vi "PH_gentec_Powermeter.PC Set Statistics Config.vi"(0 "VI in":refnum<vi>, 2 "Data Sampling Settings":T1={"Sample Rate"=0, "Sample Rate Unit"=1, "Sample Period"=0, "Sample Period Unit"=0, "Total Duration"=0, "Total Duration Unit"=0, "Time Stamp"=0} {"Time Stamp" items=["Off", "On"]; "Total Duration Unit" items=["Period", "Seconds", "Minutes", "Hours", "Days", "Weeks", "Continuous", "# of Points"]; "Total Duration" max=300 step=1; "Sample Period Unit" items=["Seconds", "Minutes", "Hours", "Days", "Weeks", "Pulses"]; "Sample Rate Unit" items=["per Second", "per Minute", "per Hour", "per Day", "% pulses"]; "Sample Rate" max=300 step=1}, 5 "error in (no error)":errorcluster) -> (14 "VI out":refnum<vi>, 19 "error out":errorcluster)   [LabVIEW 2014, in "PH_gentec_Powermeter.lvlib"]
uses:
  PH_gentec_Powermeter.lvlib
  instr.lib/gentec-SOLO-PE/Driver/Type Defs/gentec-SOLO-PE.Data Sampling Settings.ctl
  instr.lib/gentec-SOLO-PE/gentec-SOLO-PE - Driver.lvlib
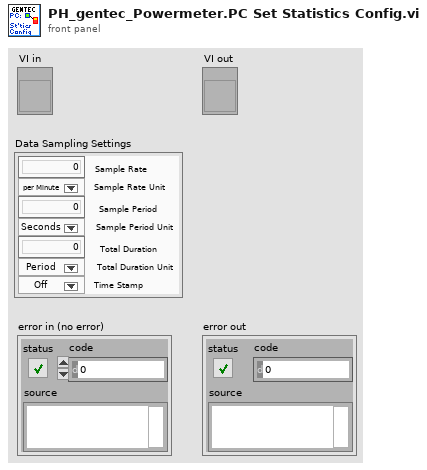
[diagram p1: front panel]
types:
  T1 = typedef "gentec-SOLO-PE - Driver.lvlib/gentec-SOLO-PE.Data Sampling Settings.ctl" = cluster{"Sample Rate":u32, "Sample Rate Unit":u32, "Sample Period":u32, "Sample Period Unit":u32, "Total Duration":u32, "Total Duration Unit":u32, "Time Stamp":u32}
  T2 = typedef "PH_gentec_Powermeter.lvlib/PH_gentec_Powermeter.i attribute.ctl" = cluster{"GUI References":cluster{"delete":refnum<vi>, "start stop Statistics":refnum<vi>, "Statistic Data":refnum<vi>, "Configuration Values":refnum<vi>, "Set Zero":refnum<vi>, "Data Sampling Settings":refnum<vi>, "Wanted Sets":refnum<vi>, "Current Sets":refnum<vi>}, "Start Stop Statistics":bool, "Wanted Sets":T3, "Current Sets":T3}
  T3 = typedef "PH_gentec_Powermeter.lvlib/PH_gentec_Powermeter.Sets.ctl" = cluster{"Data Sampling Settings":T1, "Set Zero":bool}
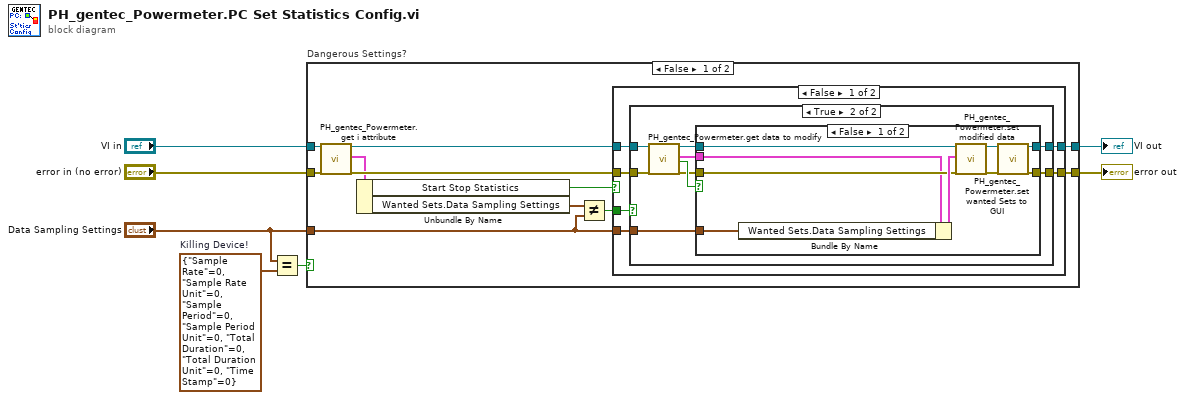
[diagram p0: block diagram]
diagram:
  w2 = T1 {"Sample Rate"=0, "Sample Rate Unit"=0, "Sample Period"=0, "Sample Period Unit"=0, "Total Duration"=0, "Total Duration Unit"=0, "Time Stamp"=0}  # Killing Device!
  n1 = Equal?(x="Data Sampling Settings", y=w2) -> (x = y?=w1:bool)
  n2 = case "Dangerous Settings?" shown="False" w1 {
    tunnel: "error in (no error)" -> [w18 w49]
    tunnel: "VI in" -> [w16 w50]
    tunnel: [w10 w50] -> w5
    tunnel: [w9 w49] -> w4
    tunnel: "Data Sampling Settings" -> [w8 _]
    frame False {
      n3 = call "PH_gentec_Powermeter.get i attribute.vi"("i ref in"=w16, "error in (no error)"=w18) -> ("i ref out"=w15:refnum<vi>, "i attribute"=w14:T2, "error out"=w17:errorcluster)  [unwired: 15 in]
      n4 = Unbundle By Name(w14) -> ("Start Stop Statistics"=w11:bool, "Wanted Sets.Data Sampling Settings"=w13:T1)
      n5 = Not Equal?(x=w13, y=w8) -> (x != y?=w12:bool)
      n6 = case shown="False" w11 {
        tunnel: w17 -> [w24 w47]
        tunnel: w15 -> [w23 w48]
        tunnel: w8 -> [w22 _]
        tunnel: w12 -> [w21 _]
        tunnel: [w20 w48] -> w10
        tunnel: [w19 w47] -> w9
        frame False {
          n7 = case shown="True" w21 {
            tunnel: [w25 w35] -> w19
            tunnel: [w26 w34] -> w20
            tunnel: w24 -> [w25 w29]
            tunnel: w23 -> [w26 w28]
            tunnel: w22 -> [_ w27]
            frame False {
            }
            frame True {
              n8 = call "PH_gentec_Powermeter.get data to modify.vi"("i ref in"=w28, "error in (no error)"=w29) -> ("i ref out"=w31:refnum<vi>, "i attribute"=w32:T2, "timed out"=w33:bool, "error out"=w30:errorcluster)  [unwired: 14 in]
              n9 = case shown="False" w33 {
                tunnel: w30 -> [w42 w45]
                tunnel: [w36 w45] -> w35
                tunnel: w31 -> [w44 w46]
                tunnel: [w38 w46] -> w34
                tunnel: w32 -> [w40 _]
                tunnel: w27 -> [w41 _]
                frame False {
                  n10 = Bundle By Name(cluster=w40, "Wanted Sets.Data Sampling Settings"=w41) -> (w43:T2)
                  n11 = call "PH_gentec_Powermeter.set modified data.vi"("i ref in"=w44, "i attribute"=w43, "error in (no error)"=w42) -> ("i ref out"=w39:refnum<vi>, "error out"=w37:errorcluster)  [unwired: 15 in]
                  n12 = call "PH_gentec_Powermeter.set wanted Sets to GUI.vi"("i ref in"=w39, "error in"=w37) -> ("i ref out"=w38:refnum<vi>, "error out"=w36:errorcluster)  [unwired: 16 in]
                }
                frame True {
                }
              }
            }
          }
        }
        frame True {
        }
      }
    }
    frame True {
    }
  }
  "error out" <- w4
  "VI out" <- w5
